vi "plunge_mode_scaled_test.vi"() -> ()   [LabVIEW 2019]
uses:
  <userlib>/Haptic Prog Interface/Haptic Prog Interface.lvlib
panel:
  out "Zthresh (m)":dbl
  in  "Fine Adj":dbl=1.0
  in  "Rough Adj.":dbl
  out "force":dbl
  out "Z Write (m) 2":dbl
  in  "Z Write?":bool
  in  "Save":bool
  in  "# Sample Points":i32=16384
  out "Signal value":sgl format="%#_6p"
  out "Z Write (m)":dbl
  in  "Upper Limit (mm)":dbl=50.0
  in  "Lower Limit (mm)":dbl=-40.0
  in  "Upper Limit (nm)":dbl=80.0
  in  "Lower Limit (nm)":dbl=79.0
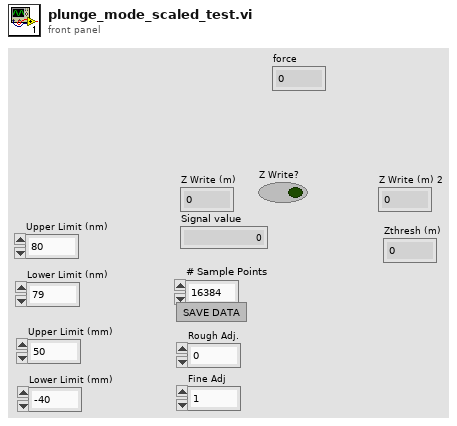
[diagram p1: front panel]
types:
  T1 = cluster{"Fx (N)":dbl, "Fy (N)":dbl, "Fz (N)":dbl}
  T2 = cluster{"x (mm)":dbl, "y (mm)":dbl, "z (mm)":dbl}
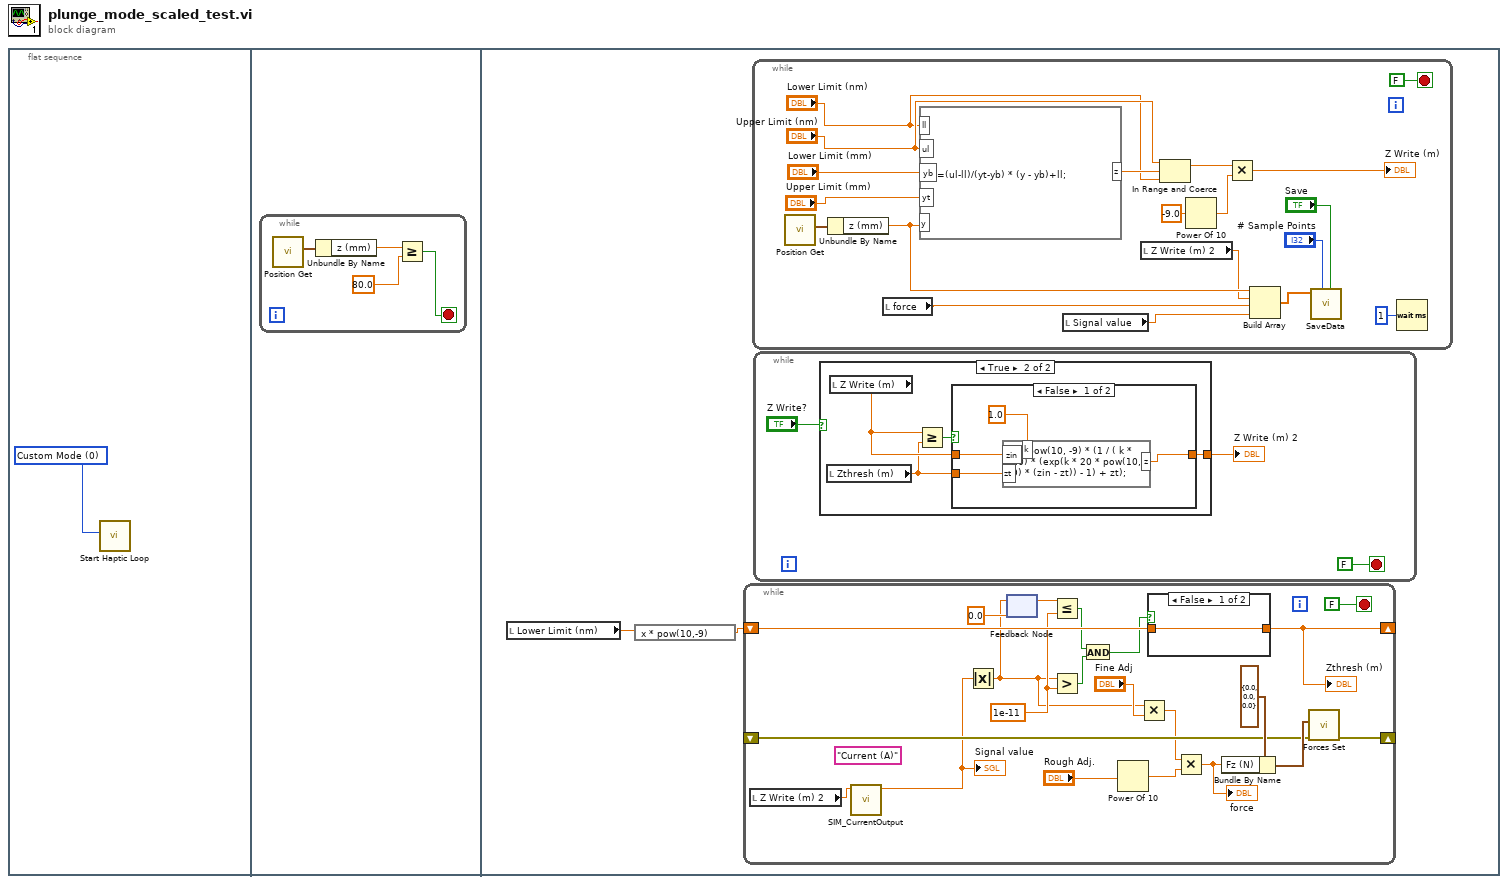
[diagram p0: block diagram]
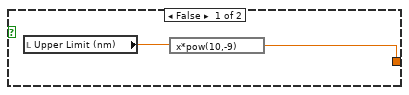
[diagram p2: hidden frame]
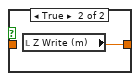
[diagram p4: hidden frame]
diagram:
  n1 = flat-sequence {
    frame #0 {
      w1 = u16 0 items=["Custom Mode", "Read Mode", "Write Mode"] ("Mode Selection")
      n2 = call <userlib>:"Start Haptic Loop.vi"("Mode Selection"=w1) -> ()  [unwired: 10 in, 1 out]
    }
    frame #1 {
      n3 = while {
        stop <- w4 stop-if-true
        n4 = call <userlib>:"Position Get.vi"() -> ("Position"=w3:T2)  [unwired: 10 in, 1 out]
        n5 = Unbundle By Name(w3) -> ("z (mm)"=w2:dbl)
        n6 = Greater Or Equal?(x=w2, y=80.0) -> (x >= y?=w4:bool)
      }
    }
    frame #2 {
      n7 = local read "Lower Limit (nm)"() -> (w7:dbl)
      n8 = expression code="x * pow(10,-9)"(w7) -> (w6:dbl)
      n9 = while {
        shift-right: [w39] -> _
        shift-left: _ -> [w38]
        shift-right: [w33] -> _
        shift-left: w6 -> [w32]
        stop <- FALSE stop-if-true
        w27 = 1e-11 ("y")
        (unwired) "Current (A)" ("Signal Name")
        n10 = local read "Z Write (m) 2"() -> (w22:dbl)
        n11 = call "SIM_CurrentOutput.vi"("zin (m)"=w22) -> ("Current Out (A)"=w23:dbl)  [unwired: 10 in]
        "Signal value" <- w23
        n12 = Absolute Value(x=w23) -> (abs(x)=w24:dbl)
        n13 = feedback-in #1(w24) -> ()
        n14 = feedback #1(sgl 0.0 ("Measurement value")) -> (w28:dbl)
        n15 = Less Or Equal?(x=w28, y=w27) -> (x <= y?=w29:bool)
        n16 = Greater?(x=w24, y=w27) -> (0:w26:bool)
        n17 = And(x=w29, y=w26) -> (x .and. y?=w31:bool)
        n18 = Power Of 10(x="Rough Adj.") -> (10^x=w36:dbl)
        n19 = Multiply(x=w24, y="Fine Adj") -> (x*y=w35:dbl)
        n20 = case shown="False" w31 {
          tunnel: [w43 w44] -> w33
          tunnel: w32 -> [w43 _]
          frame False {
          }
          frame True {
            n21 = local read "Z Write (m)"() -> (w44:dbl)
          }
        }
        "Zthresh (m)" <- w33
        n22 = Multiply(x=w35, y=w36) -> (x*y=w25:dbl)
        "force" <- w25
        n23 = Bundle By Name(cluster=T1 {"Fx (N)"=0.0, "Fy (N)"=0.0, "Fz (N)"=0.0} ("Force (N)"), "Fz (N)"=w25) -> (w40:T1)
        n24 = call <userlib>:"Forces Set.vi"("error in (no error)"=w38, "Force (N)"=w40) -> ("error out"=w39:errorcluster)  [unwired: 9 in]
      }
      n25 = while {
        stop <- FALSE stop-if-true
        n26 = call <userlib>:"Position Get.vi"() -> ("Position"=w49:T2)  [unwired: 10 in, 1 out]
        n27 = Unbundle By Name(w49) -> ("z (mm)"=w48:dbl)
        n28 = local read "force"() -> (w46:dbl)
        n29 = formula code="z =(ul-ll)/(yt-yb) * (y - yb)+ll;"("ll"="Lower Limit (nm)", "ul"="Upper Limit (nm)", "yb"="Lower Limit (mm)", "yt"="Upper Limit (mm)", "y"=w48) -> ("z"=w59:dbl)
        n30 = local read "Signal value"() -> (w52:sgl)
        n31 = local read "Z Write (m) 2"() -> (w47:dbl)
        n32 = In Range and Coerce(upper limit="Upper Limit (nm)", x=w59, lower limit="Lower Limit (nm)") -> (coerced(x)=w55:dbl)  [unwired: 1 out]
        n33 = Power Of 10(x=-9.0) -> (10^x=w60:dbl)
        n34 = Multiply(x=w55, y=w60) -> (x*y=→"Z Write (m)":dbl)
        n35 = Build Array(w48, w47, w46, w52) -> (w51:dbl[])
        n36 = call "SaveData.vi"("Save"="Save", "# Sample Points"="# Sample Points", "Data"=w51) -> ()  [unwired: 9 in]
        n37 = Wait (ms)(milliseconds to wait=u32 1) -> ()  [unwired: 1 out]
      }
      n38 = while {
        stop <- FALSE stop-if-true
        n39 = case shown="True" "Z Write?" {
          tunnel: [w11 w15] -> w8
          frame False {
            n40 = local read "Upper Limit (nm)"() -> (w12:dbl)
            n41 = expression code="x*pow(10,-9)"(w12) -> (w11:dbl)
          }
          frame True {
            n42 = local read "Zthresh (m)"() -> (w13:dbl)
            n43 = local read "Z Write (m)"() -> (w14:dbl)
            n44 = Greater Or Equal?(x=w14, y=w13) -> (x >= y?=w16:bool)
            n45 = case shown="False" w16 {
              tunnel: w14 -> [w20 w21]
              tunnel: [w18 w21] -> w15
              tunnel: w13 -> [w19 _]
              frame False {
                n46 = formula code="z =pow(10, -9) * (1 / ( k * 20) * (exp(k * 20 * pow(10, 9) * (zin - zt)) - 1) + zt);"("zt"=w19, "zin"=w20, "k"=1.0 ("input variable")) -> ("z"=w18:dbl)
              }
              frame True {
              }
            }
          }
        }
        "Z Write (m) 2" <- w8
      }
    }
  }
